vi "Introduce.vi"(8 "Error In":errorcluster, 11 "Jedi in":refnum<class "Jedi.lvclass">) -> (0 "Error Out":errorcluster, 3 "Jedi out":refnum<class "Jedi.lvclass">)   [LabVIEW 2020, in "Jedi.lvclass"]
doc: "Show name of Jedi in prompt message for user. Comments in Polish."
uses:
  Jedi.lvclass
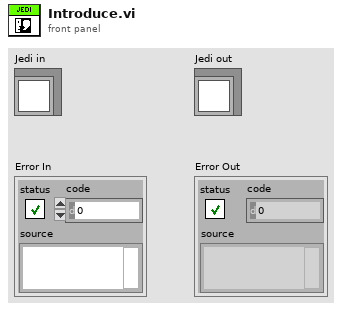
[diagram p1: front panel]
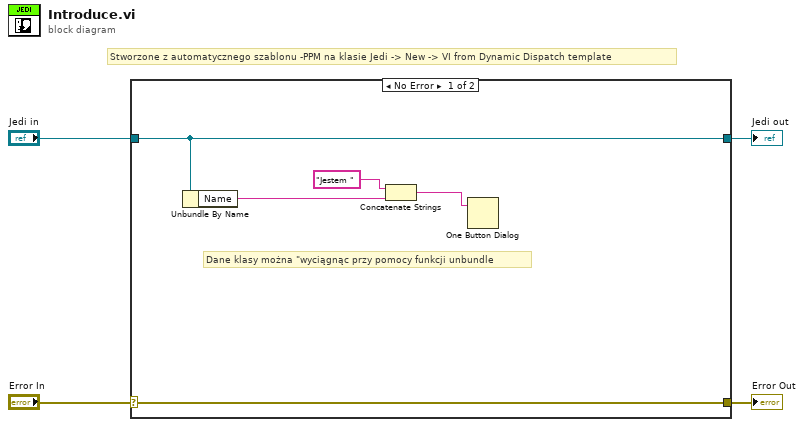
[diagram p0: block diagram]
diagram:
  # "Stworzone z automatycznego szablonu -PPM na klasie Jedi -> New -> VI from Dynamic Dispatch template"
  n1 = case shown="No Error" "Error In" {
    selector: "Error In" -> [w9 w11]
    tunnel: [w9 w11] -> w3
    tunnel: [w8 w10] -> w1
    tunnel: "Jedi in" -> [w8 w10]
    frame No Error {
      # "Dane klasy można \"wyciągnąc przy pomocy funkcji unbundle"
      n2 = Unbundle By Name(w8) -> ("Name"=w6:string)
      n3 = Concatenate Strings("Jestem ", w6) -> (w5:string)
      n4 = One Button Dialog(message=w5) -> ()  [unwired: 1 in, 1 out]
    }
    frame Error {
    }
  }
  "Error Out" <- w3
  "Jedi out" <- w1
